vi "find channel by name.vi"(10 "channel name":string, 11 "bin datalogger configuration in":refnum<class "Binary datalogger configuration.lvclass">) -> (2 "channel":refnum<class "TBM channel.lvclass">, 3 "bin datalogger configuration out":refnum<class "Binary datalogger configuration.lvclass">)   [LabVIEW 2013, in "Binary datalogger configuration.lvclass"]
uses:
  Binary datalogger configuration.lvclass
  <vilib>/NI/Tag Bus Module Framework/channel/TBM channel.lvclass
  <vilib>/NI/Tag Bus/tag/tag descriptor.lvclass/tag descriptor.ctl
  <vilib>/NI/Tag Bus/tag/read tag name.vi
  <vilib>/NI/Tag Bus/tag/tag descriptor.lvclass
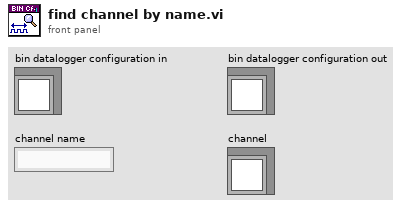
[diagram p1: front panel]
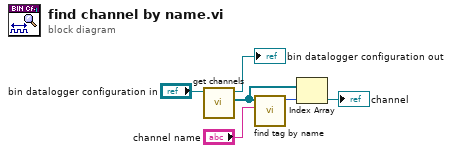
[diagram p0: block diagram]
diagram:
  n1 = call-dynamic "get channels.vi"("module configuration in"="bin datalogger configuration in") -> ("channels"=w4:refnum<class "TBM channel.lvclass">[], "module configuration out"=→"bin datalogger configuration out":refnum<class "Binary datalogger configuration.lvclass">)  [unwired: 9 in]
  n2 = call <vilib>:"find tag by name.vi"("name"="channel name", "tags in"=w4) -> ("index"=w5:i32)  [unwired: 9 in]
  n3 = Index Array(array=w4, index=w5) -> (element=→"channel":refnum<class "TBM channel.lvclass">)
